vi "Package Typed Message.vi"(8 "error in (no error)":errorcluster, 11 "Group in":refnum<class "Group.lvclass">) -> (0 "error out":errorcluster, 2 "Data Msg":refnum<class "Message.lvclass">, 3 "Group out":refnum<class "Group.lvclass">)   [LabVIEW 2020, in "Vecto.lvlib" / "Group.lvclass"]
uses:
  Group.lvclass
  C:/dev/lv20CE/relink/lv-vecto/Vecto/GroupAbstract/GroupAbstract.lvclass
  lv-protoc/LV-Proto/Message/Message.lvclass
  GroupAbstract/GroupAbstract.lvclass/GroupAbstract.ctl
  Group.lvclass/Group.ctl
  proto/GroupData/Data.ctl
  Group Config/Group Config.lvclass/Group Config.ctl
  proto/GroupData/Class/Msg.lvclass/Msg.ctl
  proto/GroupData/Class/Msg.lvclass
  C:/dev/lv20CE/relink/lv-protoc/LV-Proto/Message/Message.lvclass
  proto/GroupData/GroupData.lvlib
  Vecto.lvlib
  Group Config/Group Config.lvclass
  GroupAbstract/GroupAbstract.lvclass
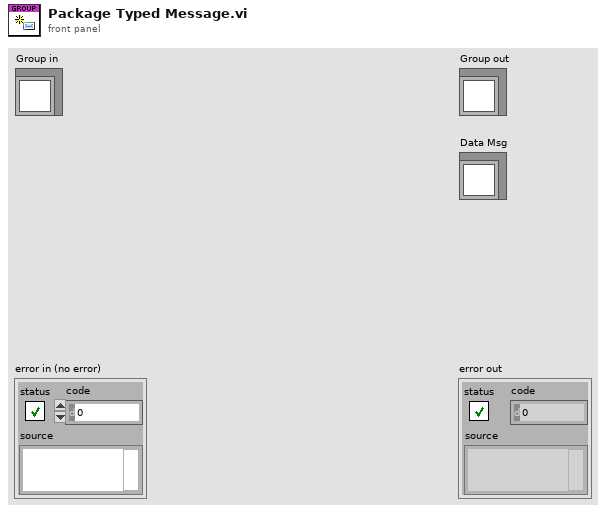
[diagram p1: front panel]
types:
  T1 = typedef "GroupData.lvlib/Data.ctl" = cluster{"group_name":string, "data_timestamp":i64, "scaled_data":dbl[], "raw_data":dbl[]}
  T2 = typedef "Vecto.lvlib/Group.lvclass/Ref.ctl" = cluster{"Scaled":dbl[], "Timestamp":dbl[], "Raw":dbl[]}
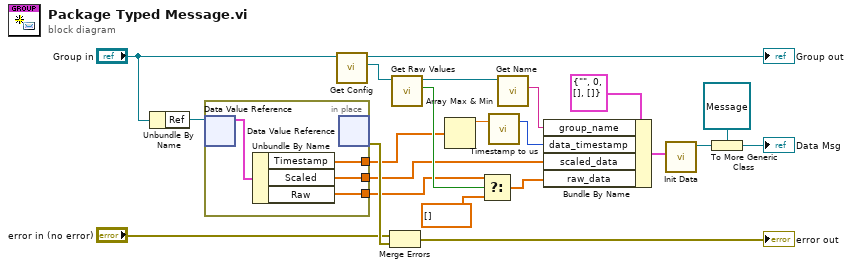
[diagram p0: block diagram]
diagram:
  n1 = Unbundle By Name("Group in") -> ("Ref"=w19:refnum<data-value>)
  n2 = in-place {
    in-place-border: [w25] -> w6
    in-place-border: [w24] -> w7
    in-place-border: [w23] -> w5
    n3 = in-place-dvr #1(w19) -> (w26:T2)  [unwired: 1 out]
    n4 = Unbundle By Name(w26) -> ("Timestamp"=w24:dbl[], "Scaled"=w25:dbl[], "Raw"=w23:dbl[])
    n5 = in-place-dvr #1() -> (w22:errorcluster)  [unwired: 1 in, 1 out]
  }
  n6 = call "Get Config.vi"("GroupAbstract in"="Group in") -> ("Config"=w3:refnum<class "Group Config.lvclass">, "GroupAbstract out"=→"Group out":refnum<class "Group.lvclass">)  [unwired: 8 in, 1 out]
  n7 = Merge Errors("error in (no error)", w22) -> (→"error out":errorcluster)
  n8 = call "Get Raw Values.vi"("Group Config in"=w3) -> ("Raw Values"=w12:bool, "Group Config out"=w11:refnum<class "Group Config.lvclass">)  [unwired: 8 in, 1 out]
  n9 = Array Max & Min(array=w7) -> (max value=w17:dbl)  [unwired: 3 out]
  n10 = Select(t=w5, s=w12, f=dbl[] []) -> (s? t:f=w13:dbl[])
  n11 = call "Timestamp to us.vi"("Timestamp"=w17) -> ("Timestamp us"=w16:i64)  [unwired: 6 in]
  n12 = call "Get Name.vi"("Group Config in"=w11) -> ("Name"=w10:string)  [unwired: 8 in, 2 out]
  n13 = Bundle By Name(cluster=T1 {"group_name"="", "data_timestamp"=0, "scaled_data"=[], "raw_data"=[]} ("GroupData"), "group_name"=w10, "data_timestamp"=w16, "scaled_data"=w6, "raw_data"=w13) -> (w9:T1)
  n14 = call "Init Data.vi"("Data"=w9) -> ("Msg out"=w8:refnum<class "Msg.lvclass">)  [unwired: 10 in]
  n15 = To More Generic Class(target class=refnum<class "Message.lvclass"> refnum ("LV-Proto.lvlib:Message.lvclass"), reference=w8) -> (generic class reference=→"Data Msg":refnum<class "Message.lvclass">)
